vi "Samples to be acquired.vi"(8 "error in (no error)":errorcluster, 10 "AOL_Globals":T1={"Imaging Protocol"=enum."AOL Z-Stack", "Number of POI"=0, "Number of Miniscans"=0, "Number of Trials"=0, "Number of Cycles "=0, "# Averaged Frames"=0, "Laser power (%)"=0, "Pockels (V)"=0.0, "Acquisition Length (sec)"=0.0, "Fill time (us)"=0.0, "POI Dwell time (us)"=0.0, "Miniscan Dwell time per pixel (us)"=0.0, "PMT 1"=0.0, "PMT 2"=0.0, "Back Apperture (mA)"=200.0, "Frame Size"=0, "Center Frequency"=0.0, "Field of View (um)"=175.0, "Field of View (norm)"=0.0, "DwellTime (us)"=0.0, "Ref Dwell Time (us)"=0.0, "Wavelength (nm)"=0.0, "Zoom"=0.0, "AOL Z"=0.0, "AOL Mode"=enum."Raster", "GridXY"=0.0, "GridZ"=0.0, "TriggerPeriod (sec)"=0.0, "Number of Pixels in Miniscan"=0, "Experiment folder path"=path "", "X centre"=0.0, "Y centre"=0.0, "Angle (degrees)"=0.0, "Angle Xs (degrees)"=0.0, "Angle Ys (degrees)"=0.0, "Plane Mode"=0, "Threshold"=[], "Regenerate Chirps"=FALSE, "Rectangle ROI length (pixels)"=0, "Rectangle ROI height (pixels)"=0, "AOD fill"=4900, "StartupDelay"=0, "Samples Wait after Trigger"=5080, "Slip Cycle"=600000, "Add Cycle"=TRUE, "Functional Mode"=enum."Point", "Z Start"=0.0, "Z Stop"=0.0, "# Planes"=0, "Total Pixels"=0, "Variable Miniscan Pixels"=[], "Use Variable Length"=FALSE, "Use Variable Resolution"=FALSE, "Laser power (%) at Z Start"=0, "Laser power (%) at Z Stop"=0, "Ref Z Step"=0} {"Angle Ys (degrees)" format="%#.6g"; "Angle Xs (degrees)" format="%#.6g"; "Plane Mode" items=["XY Plane", "XZ Plane", "YZ Plane", "arbitraryplane"]; "Frame Size" items=["100X100"=100, "128X128"=128, "200X200"=200, "256X256"=256, "512X512"=512, "1024x1024"=1024, "2048x2048"=2048]; "Back Apperture (mA)" format="%#.6g"; "Pockels (V)" format="%#.6g"; "PMT 2" format="%#.6g"; "PMT 1" format="%#.6g"; "Angle (degrees)" format="%#.6g"; "POI Dwell time (us)" format="%#.6g"}) -> (0 "error out":errorcluster, 1 "Number of Ref samples to be acquired":u32, 2 "Number of samples to be acquired (points in frame x Ch. x Av.)":u64)   [LabVIEW 2020]
uses:
  Typedefs/Controls/AOL_Globals.ctl
  Typedefs/Imaging Protocols enum.ctl
  Typedefs/Frame Size.ctl
  Typedefs/AOL modes.ctl
  Typedefs/Plane Mode.ctl
  Typedefs/Functional Mode.ctl
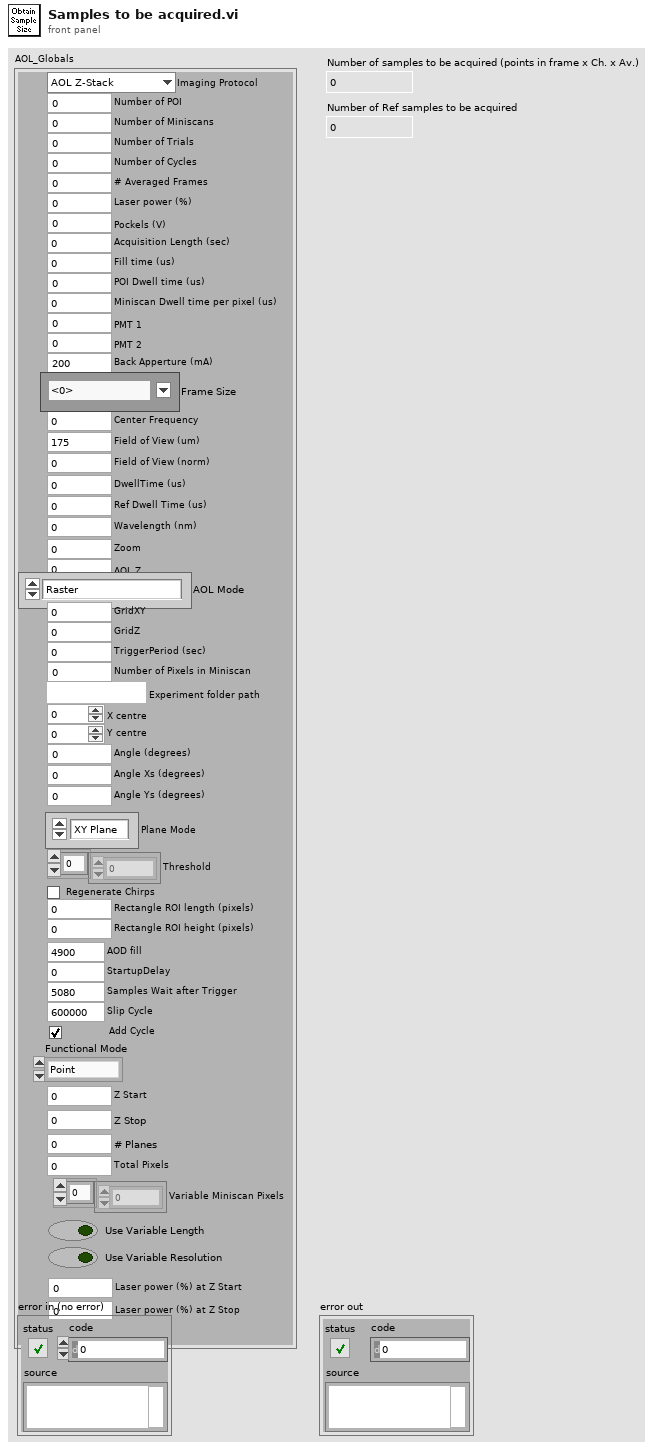
[diagram p1: front panel]
types:
  T1 = typedef "AOL_Globals.ctl" = cluster{"Imaging Protocol":T2, "Number of POI":u16, "Number of Miniscans":u16, "Number of Trials":u16, "Number of Cycles ":u64, "# Averaged Frames":u16, "Laser power (%)":u8, "Pockels (V)":dbl, "Acquisition Length (sec)":dbl, "Fill time (us)":dbl, "POI Dwell time (us)":dbl, "Miniscan Dwell time per pixel (us)":dbl, "PMT 1":dbl, "PMT 2":dbl, "Back Apperture (mA)":dbl, "Frame Size":T3, "Center Frequency":dbl, "Field of View (um)":dbl, "Field of View (norm)":dbl, "DwellTime (us)":dbl, "Ref Dwell Time (us)":dbl, "Wavelength (nm)":dbl, "Zoom":dbl, "AOL Z":dbl, "AOL Mode":T4, "GridXY":dbl, "GridZ":dbl, "TriggerPeriod (sec)":dbl, "Number of Pixels in Miniscan":u16, "Experiment folder path":path, "X centre":dbl, "Y centre":dbl, "Angle (degrees)":dbl, "Angle Xs (degrees)":dbl, "Angle Ys (degrees)":dbl, "Plane Mode":T5, "Threshold":u16[], "Regenerate Chirps":bool, "Rectangle ROI length (pixels)":u16, "Rectangle ROI height (pixels)":u16, "AOD fill":u16, "StartupDelay":i32, "Samples Wait after Trigger":u16, "Slip Cycle":u32, "Add Cycle":bool, "Functional Mode":T6, "Z Start":dbl, "Z Stop":dbl, "# Planes":i32, "Total Pixels":i32, "Variable Miniscan Pixels":u16[], "Use Variable Length":bool, "Use Variable Resolution":bool, "Laser power (%) at Z Start":u8, "Laser power (%) at Z Stop":u8, "Ref Z Step":i8}
  T2 = typedef "Imaging Protocols enum.ctl" = enum16{"AOL Z-Stack", "Motor Z Stack", "Parameter Sweep", "Functional Acquisition", "Single Plane Acquisition", "Volume Acquisition", "Live Imaging", "Live Plane Imaging", "Live Volume Imaging"}
  T3 = typedef "Frame Size.ctl" = u16
  T4 = typedef "AOL modes.ctl" = enum16{"Raster", "Structural", "Pointing", "Mini Scan", "Alignment"}
  T5 = typedef "Plane Mode.ctl" = u16
  T6 = typedef "Functional Mode.ctl" = enum16{"Point", "Line", "Patch", "Plane", "Volume"}
  T7 = typedef "Ref DAQ Param.ctl" = cluster{"Full Frame Size":u16, "Ref Field of View":sgl, "Ref Zoom":i8, "Ref_dwellTime":sgl, "Ref X-pixels-per-line(Npxr)":i16, "Ref Y-lines-per-image(Npyr)":i16, "Ref Z-lines-per-image":i16, "Ignore Z lines":i16, "Ref Scan Cycles":i32, "Ref threshold XY":u16, "Ref threshold Z":u16, "Ref average XY":u16, "Ref Average  Z":u16, "Proportional_scale":fxp<+,16,2>, "Integral_scale":fxp<+/-,16,12>, "Proportional_scale Z":fxp<+,16,2>, "Integral_scale Z":fxp<+/-,16,12>, "Diff_threshold":fxp<+,16,2>, "Diff_threshold _z":fxp<+,16,2>, "Sliding Average":bool, "Ref count reset enabled":bool, "Auto-centering":bool}
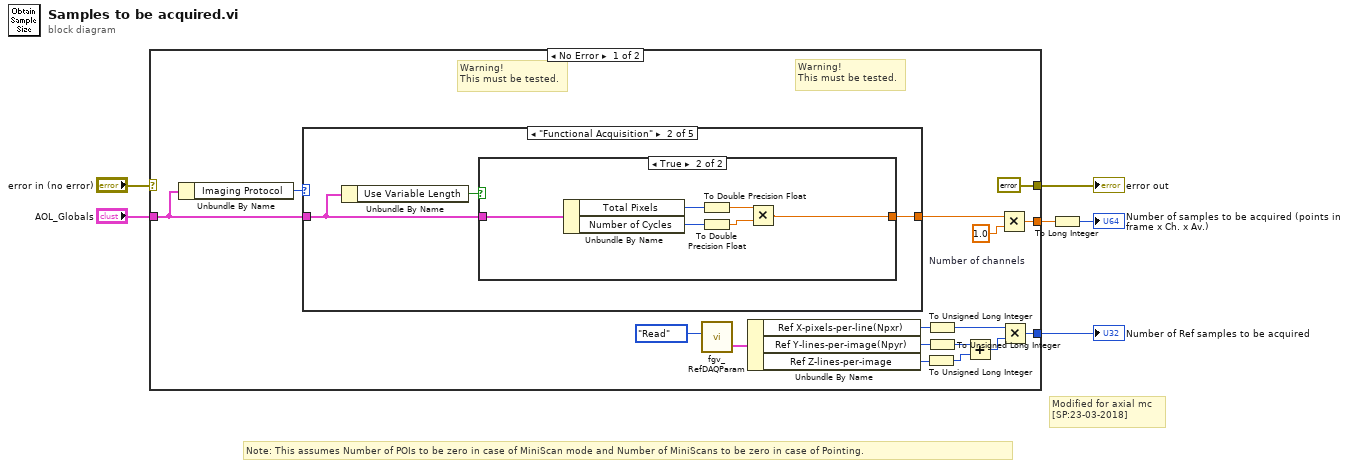
[diagram p0: block diagram]
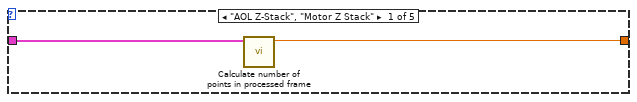
[diagram p2: hidden frame]
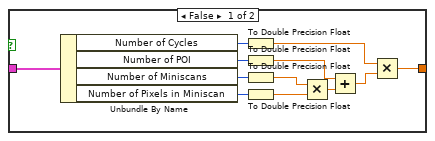
[diagram p3: hidden frame]
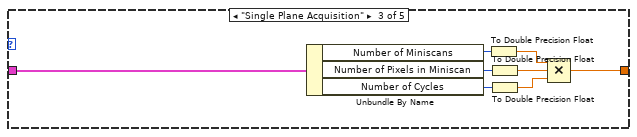
[diagram p4: hidden frame]
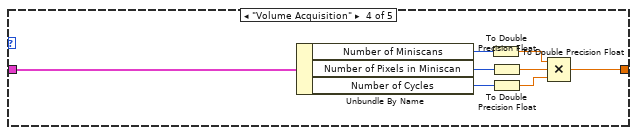
[diagram p5: hidden frame]
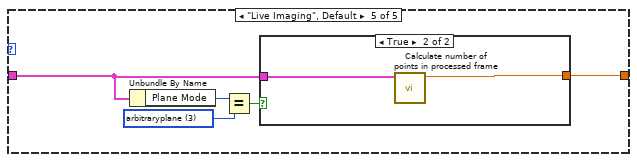
[diagram p6: hidden frame]
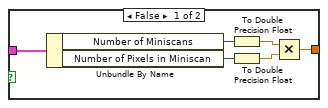
[diagram p7: hidden frame]
diagram:
  # "Modified for axial mc\n[SP:23-03-2018]"
  # "Note: This assumes Number of POIs to be zero in case of MiniScan mode and Number of MiniScans to be zero in case of Pointing."
  n1 = case shown="No Error" "error in (no error)" {
    selector: "error in (no error)" -> [_ w75]
    tunnel: "AOL_Globals" -> [w19 _]
    tunnel: [w18 _] -> w5
    tunnel: [errorcluster {"status"=FALSE, "code"=0, "source"=""} ("error IO") w75] -> w3
    tunnel: [w12 _] -> w1
    frame No Error {
      w21 = 1.0  # Number of channels
      # "Warning!\nThis must be tested."
      # "Warning!\nThis must be tested."
      n2 = Unbundle By Name(w19) -> ("Imaging Protocol"=w22:T2)
      n3 = case shown="\"Functional Acquisition\"" w22 {
        tunnel: [w23 w27 w48 w56 w66] -> w20
        tunnel: w19 -> [w24 w26 w53 w61 w65]
        frame "AOL Z-Stack", "Motor Z Stack" {
          n4 = call "Calculate number of points in processed frame.vi"("AOL_Globals"=w24) -> ("Number of points in averaged frame or single frame"=w23:dbl)  [unwired: 10 in]
        }
        frame "Functional Acquisition" {
          n5 = Unbundle By Name(w26) -> ("Use Variable Length"=w25:bool)
          n6 = case shown="True" w25 {
            tunnel: w26 -> [w39 w45]
            tunnel: [w32 w40] -> w27
            frame False {
              n7 = Unbundle By Name(w39) -> ("Number of Cycles"=w38:u64, "Number of POI"=w33:u16, "Number of Miniscans"=w36:u16, "Number of Pixels in Miniscan"=w34:u16)
              n8 = To Double Precision Float(number=w38) -> (double precision float=w37:dbl)
              n9 = To Double Precision Float(number=w33) -> (double precision float=w31:dbl)
              n10 = To Double Precision Float(number=w36) -> (double precision float=w30:dbl)
              n11 = To Double Precision Float(number=w34) -> (double precision float=w29:dbl)
              n12 = Multiply(x=w30, y=w29) -> (x*y=w35:dbl)
              n13 = Add(x=w31, y=w35) -> (x+y=w28:dbl)
              n14 = Multiply(x=w37, y=w28) -> (x*y=w32:dbl)
            }
            frame True {
              n15 = Unbundle By Name(w45) -> ("Total Pixels"=w43:i32, "Number of Cycles"=w44:u64)
              n16 = To Double Precision Float(number=w43) -> (double precision float=w42:dbl)
              n17 = To Double Precision Float(number=w44) -> (double precision float=w41:dbl)
              n18 = Multiply(x=w42, y=w41) -> (x*y=w40:dbl)
            }
          }
        }
        frame "Single Plane Acquisition" {
          n19 = Unbundle By Name(w53) -> ("Number of Miniscans"=w50:u16, "Number of Pixels in Miniscan"=w51:u16, "Number of Cycles"=w52:u64)
          n20 = To Double Precision Float(number=w50) -> (double precision float=w49:dbl)
          n21 = To Double Precision Float(number=w51) -> (double precision float=w47:dbl)
          n22 = To Double Precision Float(number=w52) -> (double precision float=w46:dbl)
          n23 = Compound Arithmetic op=MULTIPLY(w49, w47, w46) -> (w48:dbl)
        }
        frame "Volume Acquisition" {
          n24 = Unbundle By Name(w61) -> ("Number of Miniscans"=w58:u16, "Number of Pixels in Miniscan"=w59:u16, "Number of Cycles"=w60:u64)
          n25 = To Double Precision Float(number=w58) -> (double precision float=w57:dbl)
          n26 = To Double Precision Float(number=w59) -> (double precision float=w55:dbl)
          n27 = To Double Precision Float(number=w60) -> (double precision float=w54:dbl)
          n28 = Compound Arithmetic op=MULTIPLY(w57, w55, w54) -> (w56:dbl)
        }
        frame "Live Imaging", Default {
          w63 = T5 3 items=["XY Plane", "XZ Plane", "YZ Plane", "arbitraryplane"] ("y")
          n29 = Unbundle By Name(w65) -> ("Plane Mode"=w64:T5)
          n30 = Equal?(x=w64, y=w63) -> (x = y?=w62:bool)
          n31 = case shown="True" w62 {
            tunnel: w65 -> [w68 w74]
            tunnel: [w67 w73] -> w66
            frame False {
              n32 = Unbundle By Name(w68) -> ("Number of Miniscans"=w72:u16, "Number of Pixels in Miniscan"=w71:u16)
              n33 = To Double Precision Float(number=w72) -> (double precision float=w70:dbl)
              n34 = To Double Precision Float(number=w71) -> (double precision float=w69:dbl)
              n35 = Multiply(x=w70, y=w69) -> (x*y=w67:dbl)
            }
            frame True {
              n36 = call "Calculate number of points in processed frame.vi"("AOL_Globals"=w74) -> ("Number of points in averaged frame or single frame"=w73:dbl)  [unwired: 10 in]
            }
          }
        }
      }
      n37 = call "fgv_RefDAQParam.vi"("Function"=enum16{"Initialize", "Write", "Read"}."Read" ("Status")) -> ("RefDAQParam"=w15:T7)  [unwired: 9 in, 1 out]
      n38 = Unbundle By Name(w15) -> ("Ref X-pixels-per-line(Npxr)"=w13:i16, "Ref Y-lines-per-image(Npyr)"=w14:i16, "Ref Z-lines-per-image"=w10:i16)
      n39 = To Unsigned Long Integer(number=w10) -> (unsigned 32bit integer=w9:u32)
      n40 = To Unsigned Long Integer(number=w13) -> (unsigned 32bit integer=w11:u32)
      n41 = To Unsigned Long Integer(number=w14) -> (unsigned 32bit integer=w8:u32)
      n42 = Add(x=w8, y=w9) -> (x+y=w7:u32)
      n43 = Multiply(x=w20, y=w21) -> (x*y=w18:dbl)
      n44 = Multiply(x=w11, y=w7) -> (x*y=w12:u32)
    }
    frame Error {
    }
  }
  "error out" <- w3
  "Number of Ref samples to be acquired" <- w1
  n45 = To Long Integer(number=w5) -> (32bit integer=→"Number of samples to be acquired (points in frame x Ch. x Av.)":i32)
